vi "TorqueAndForceRead.vi"(8 "error in (no error)":errorcluster, 11 "Data Cluster":T1) -> (0 "error out":errorcluster, 1 "Array":dbl[][](array[numeric]))   [LabVIEW 2026, in "Acquisition.lvlib"]
uses:
  Acquisition.lvlib
  <vilib>/DAQmx/read.llb/DAQmx Read (Analog 1D Wfm NChan NSamp).vi
  Hardware Configuration.ctl
panel:
  out "Strain Guage Voltage":dbl
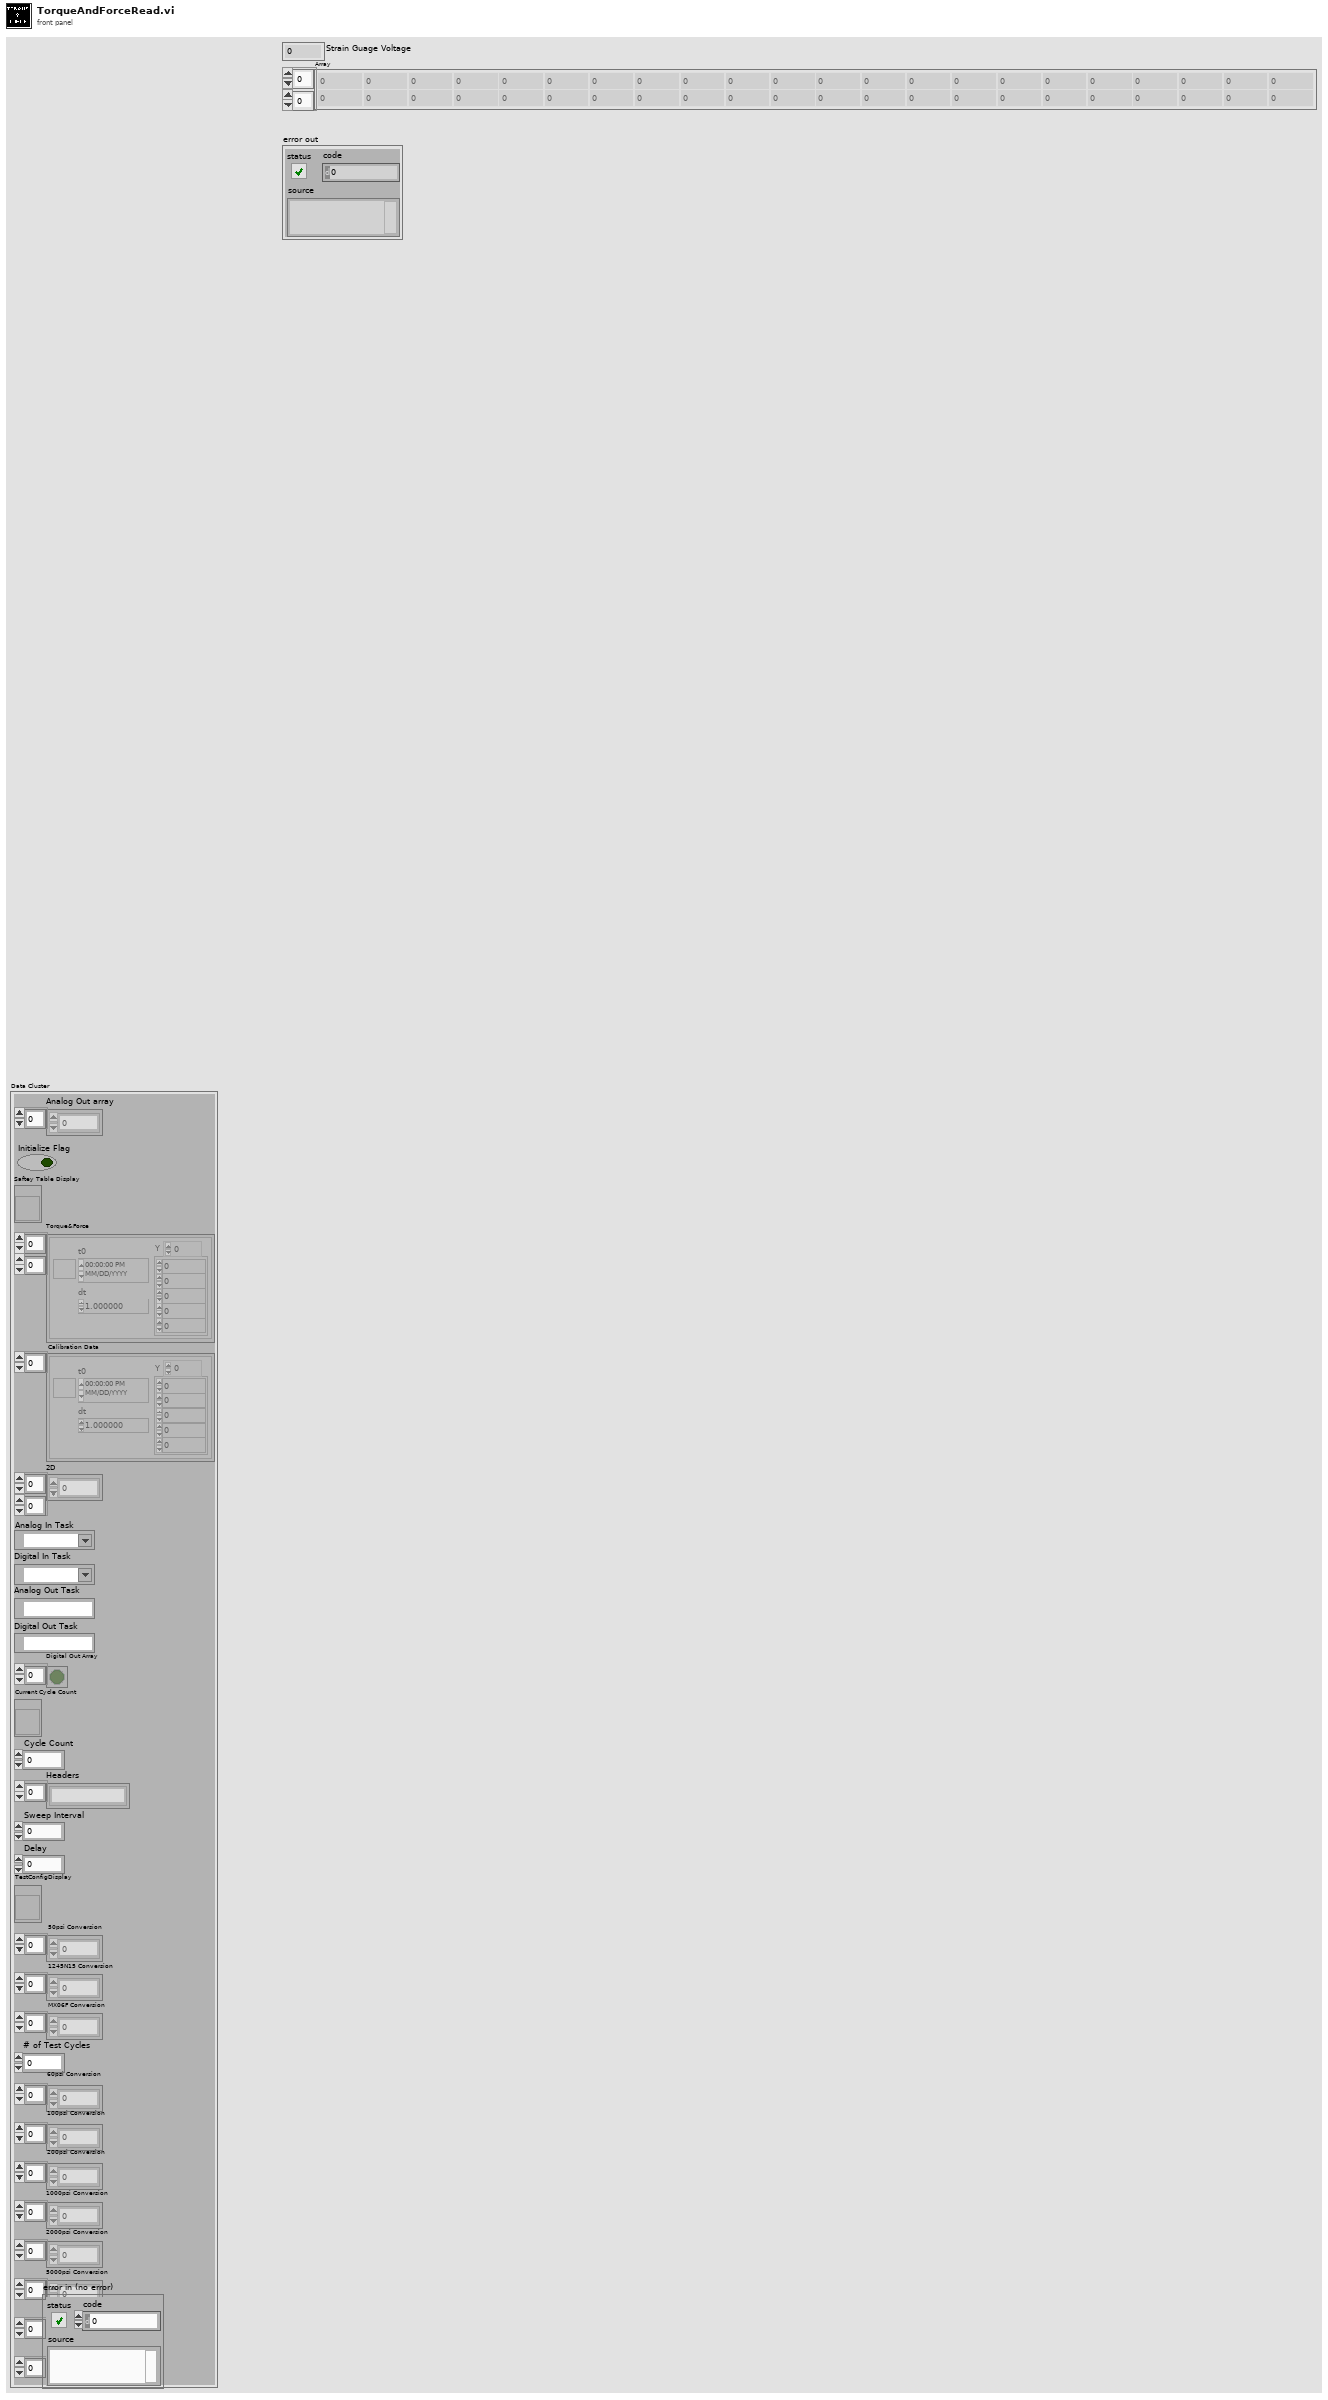
[diagram p1: front panel]
types:
  T1 = typedef "Acquisition.lvlib/Hardware Configuration.ctl" = cluster{"Analog Out array":dbl[], "Initialize Flag":bool, "Saftey Table Display":refnum<vi>, "Torque&Force":waveform(dbl)[][], "Calibration Data":waveform(dbl)[], "2D":dbl[][], "Analog In Task":refnum<k21>, "Digital In Task":refnum<k21>, "Analog Out Task":refnum<k21>, "Digital Out Task":refnum<k21>, "Digital Out Array":bool[], "Current Cycle Count":refnum<vi>, "Cycle Count":u64, "Headers":string[], "Sweep Interval":u64, "Delay":u64, "TestConfigDisplay":refnum<vi>, "50psi Conversion":dbl[], "1245N15 Conversion":dbl[], "MX06F Conversion":dbl[], "# of Test Cycles":u64, "60psi Conversion":dbl[], "100psi Conversion":dbl[], "200psi Conversion":dbl[], "1000psi Conversion":dbl[], "2000psi Conversion":dbl[], "5000psi Conversion":dbl[], "MX09F Conversion":dbl[], "MX19F Conversion":dbl[]}
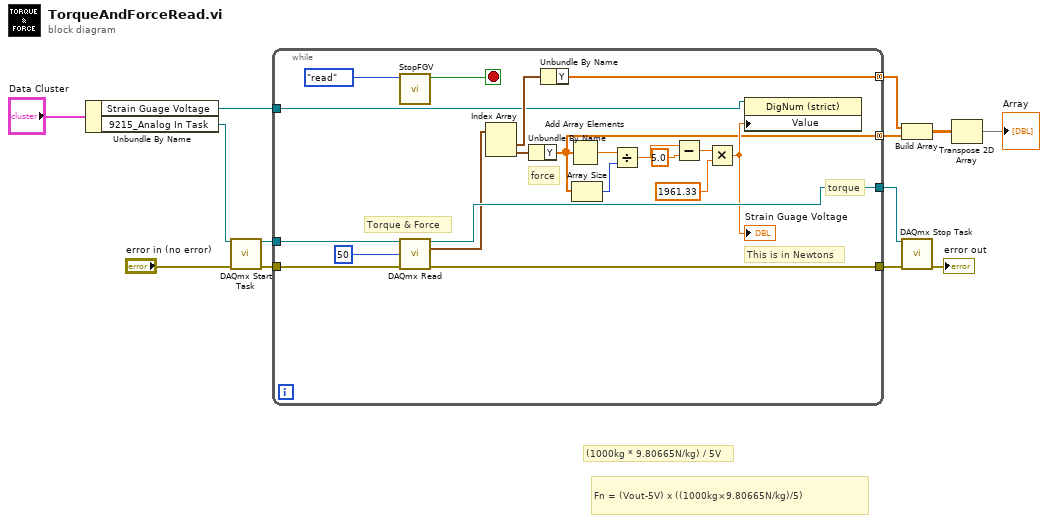
[diagram p0: block diagram]
diagram:
  # "Fn = (Vout-5V) x ((1000kg×9.80665N/kg)/5)"
  # "(1000kg * 9.80665N/kg) / 5V"
  n1 = Unbundle By Name("Data Cluster") -> ("Strain Guage Voltage"=w5:refnum<vi>, "9215_Analog In Task"=w6:refnum<k21>)
  n2 = call <vilib>:"DAQmx Start Task.vi"("task/channels in"=w6, "error in"="error in (no error)") -> ("task out"=w11:refnum<k21>, "error out"=w12:errorcluster)  [unwired: 12 in]
  n3 = while {
    tunnel: w12 -> [w33]
    tunnel: [w32] -> w9
    tunnel: w11 -> [w28]
    tunnel: [w27] -> w8
    tunnel: w5 -> [w16]
    tunnel: [w15] -> w3 mode=concatenating
    tunnel: [w14] -> w2 mode=concatenating
    stop <- w30 stop-if-true
    # "This is in Newtons"
    # "force"
    # "torque"
    # "Torque & Force"
    n4 = call "StopFGV.vi"("Enum"=enum16{"init", "write", "read"}."read") -> ("STOP Out"=w30:bool)  [unwired: 9 in, 1 out]
    n5 = call-poly <vilib>:"DAQmx Read.vi"("task/channels in"=w28, "number of samples per channel"=50, "error in"=w33) -> ("task out"=w27:refnum<k21>, "data"=w26:waveform(dbl)[], "error out"=w32:errorcluster)  [unwired: 10 in]
    n6 = Index Array(array=w26) -> (element #1=w25:waveform(dbl), element #2=w24:waveform(dbl))  [unwired: 2 in]
    n7 = Unbundle By Name(w24) -> ("Y"=w14:dbl[])
    n8 = Unbundle By Name(w25) -> ("Y"=w15:dbl[])
    n9 = Add Array Elements(numeric array=w14) -> (sum=w23:dbl)
    n10 = Array Size(array=w14) -> (size(s)=w22:i32)
    n11 = Divide(x=w23, y=w22) -> (x/y=w17:dbl)
    n12 = Subtract(x=w17, y=5.0) -> (x-y=w20:dbl)
    n13 = Multiply(x=w20, y=1961.33) -> (x*y=w21:dbl)
    "Strain Guage Voltage" <- w21
    n14 = property class="DigNum (strict)"(reference=w16, "Value"=w21) -> ()  [unwired: 1 in, 2 out]
  }
  n15 = Build Array(w3, w2) -> (w4:dbl[][])
  n16 = call <vilib>:"DAQmx Stop Task.vi"("task/channels in"=w8, "error in"=w9) -> ("error out"=→"error out":errorcluster)  [unwired: 12 in, 1 out]
  n17 = Transpose 2D Array(2D array=w4) -> (transposed array=→"Array":dbl[][])
